vi "RTS Macro Filter Defrost Cycle.vi"(0 "Refrigeration Full Data":T1, 5 "Refrigeration Core Stats Input":T2 {"Average Compressor Cycle Time (Min)" format="%0.2f"; "Average Compressor Power (W)" format="%0.2f"; "Power Start Time (sec)" format="%<%H:%M:%S>t"; "Power End time (sec)" format="%<%H:%M:%S>t"; "Average Defrost Power (W)" format="%0.2f"}, 11 "Error In":errorcluster, 12 "Average Compressor Power (Lower)":dbl=10.0 format="%#_13g") -> (4 "Refrigeration Full Data Output":T1, 6 "Refrigeration Core Stats":T2 {"Average Compressor Cycle Time (Min)" format="%0.2f"; "Average Compressor Power (W)" format="%0.2f"; "Power Start Time (sec)" format="%<%H:%M:%S>t"; "Power End time (sec)" format="%<%H:%M:%S>t"; "Average Defrost Power (W)" format="%0.2f"}, 15 "Error Out":errorcluster)   [LabVIEW 2016]
uses:
  Type Definitions/RTS Macro Refrigeration Core Stats.ctl
  Type Definitions/RTS Macro Full Data.ctl
panel:
  out "Power Compressor Run 2":cluster{dbl[], dbl[]}(graph)
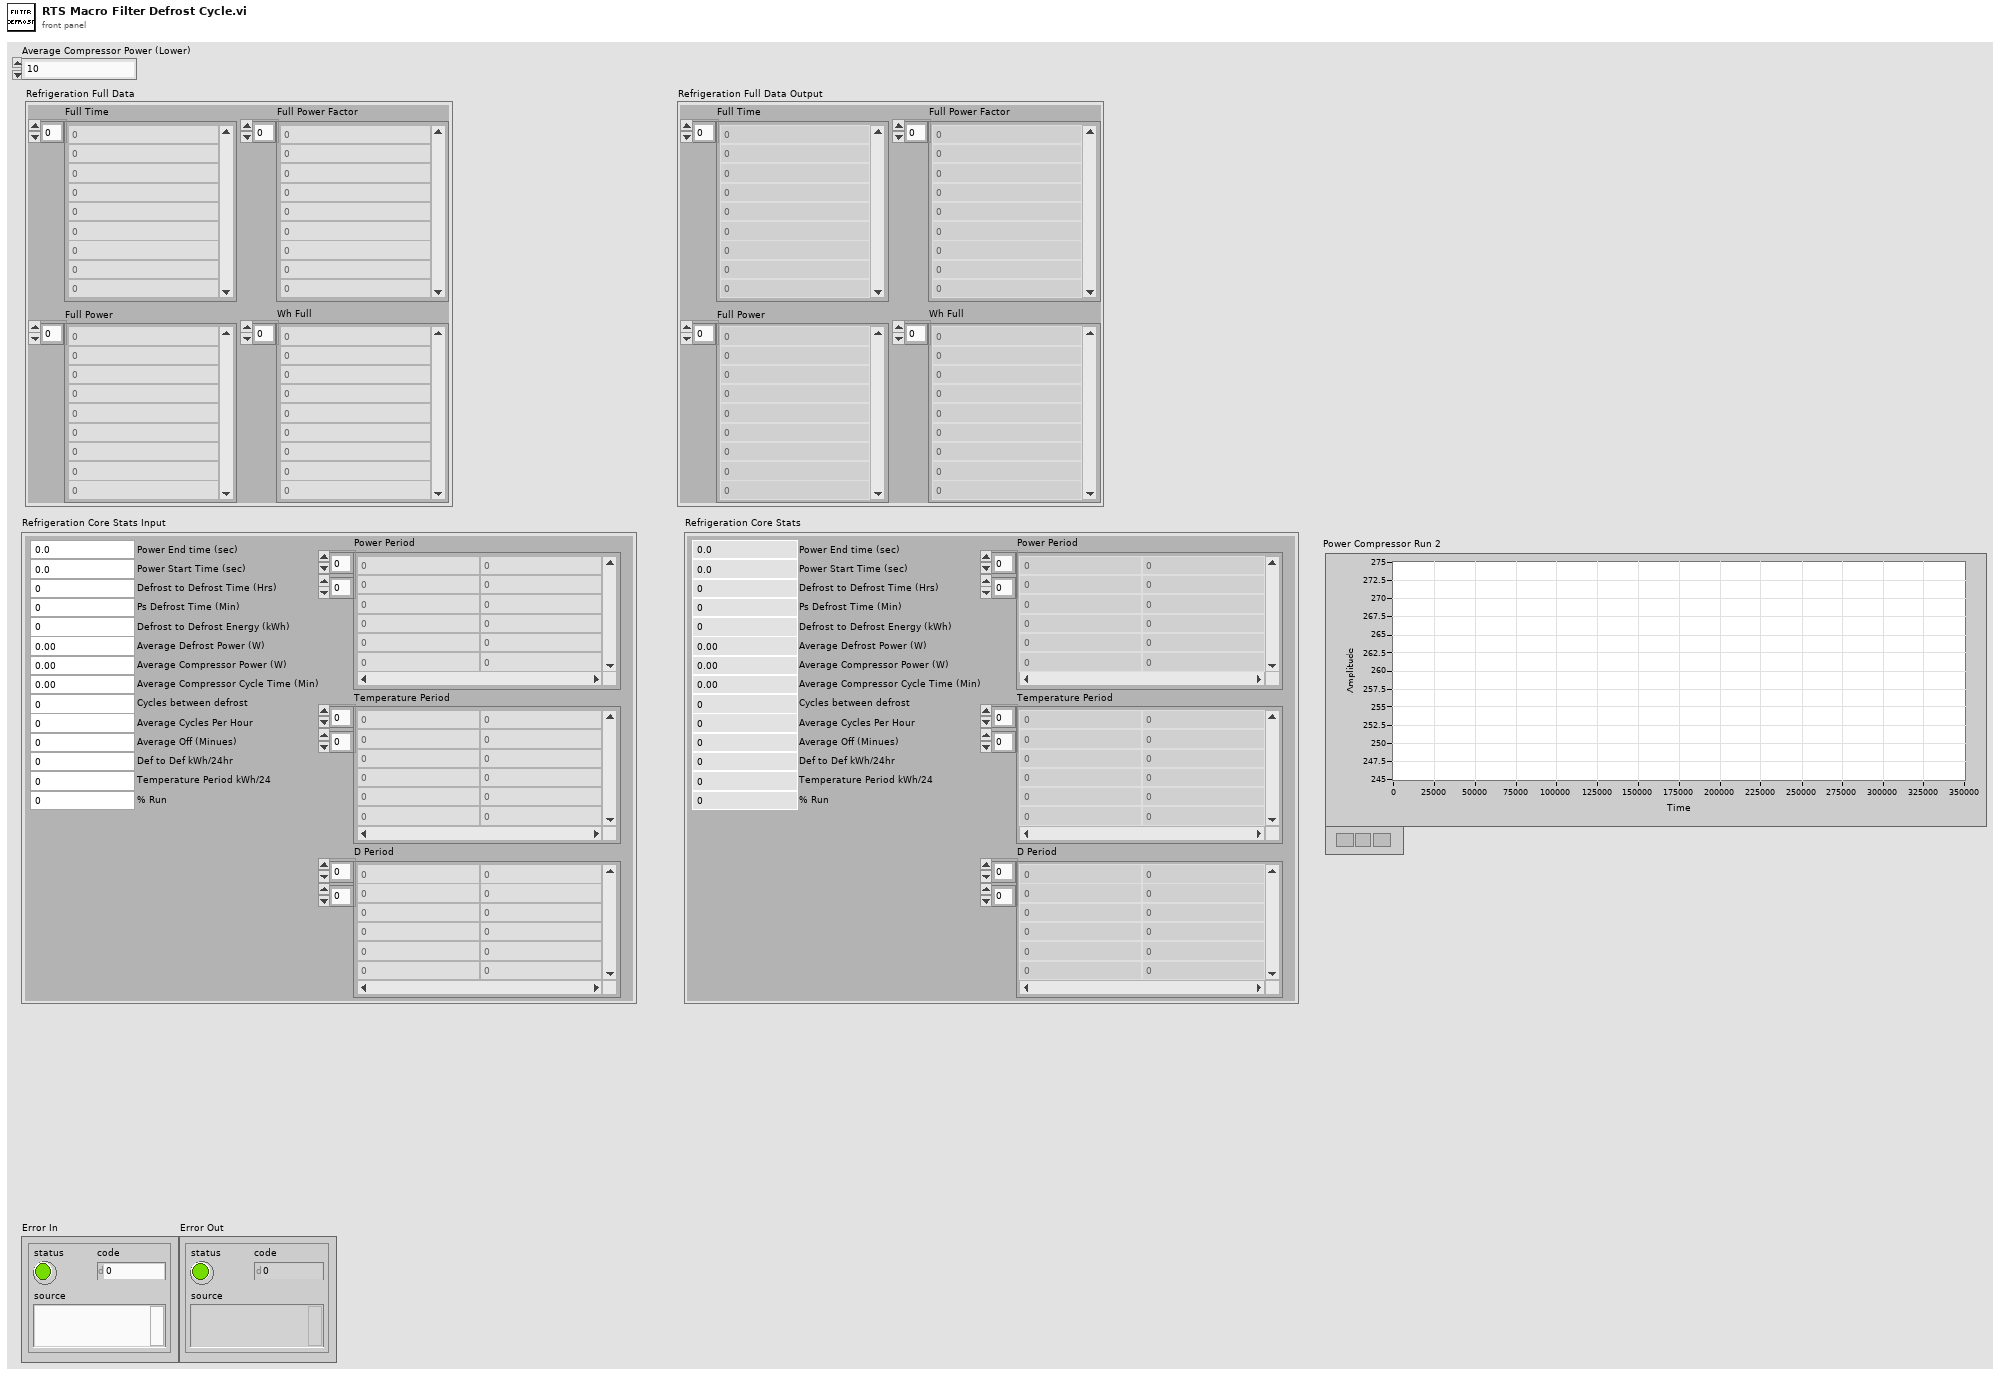
[diagram p1: front panel]
types:
  T1 = typedef "RTS Macro Full Data.ctl" = cluster{"Full Time":dbl[], "Full Power Factor":dbl[], "Full Power":dbl[], "Wh Full":dbl[]}
  T2 = typedef "RTS Macro Refrigeration Core Stats.ctl" = cluster{"Average Defrost Power (W)":dbl, "Power End time (sec)":dbl, "Power Start Time (sec)":dbl, "Defrost to Defrost Time (Hrs)":dbl, "Ps Defrost Time (Min)":dbl, "Defrost to Defrost Energy (kWh)":dbl, "Average Compressor Power (W)":dbl, "Average Compressor Cycle Time (Min)":dbl, "Power Period":dbl[][], "Cycles between defrost":i32, "Average Cycles Per Hour":dbl, "Average Off (Minues)":dbl, "Def to Def kWh/24hr":dbl, "Temperature Period kWh/24":dbl, "% Run":dbl, "Temperature Period":dbl[][], "D Period":dbl[][]}
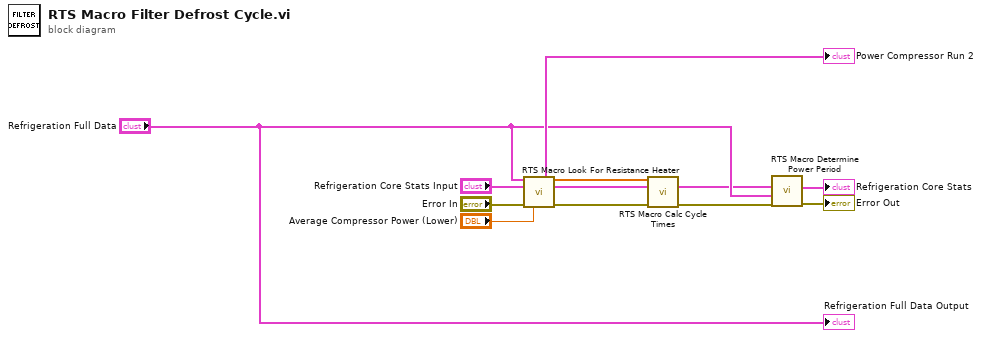
[diagram p0: block diagram]
diagram:
  n1 = call "RTS Macro Look For Resistance Heater.vi"("Refrigeration Full Data Output"="Refrigeration Full Data", "Refrigeration Core Stats Input"="Refrigeration Core Stats Input", "Error In"="Error In", "Average Compressor Power (Lower)"="Average Compressor Power (Lower)") -> ("Power Compressor Run 2"=→"Power Compressor Run 2":cluster{dbl[], dbl[]}, "Time Array"=w7:dbl[], "Refrigeration Core Stats Output"=w5:T2, "Error Out"=w9:errorcluster)  [unwired: 8 in]
  n2 = call "RTS Macro Calc Cycle Times.vi"("Time"=w7, "Refrigeration Core Stats Input"=w5, "Error In"=w9) -> ("Refrigeration Core Stats Output"=w2:T2, "Error Out"=w4:errorcluster)  [unwired: 8 in, 3 out]
  n3 = call "RTS Macro Determine Power Period.vi"("Refrigeration Core Stats Input"=w2, "Refrigeration Full Data"="Refrigeration Full Data", "Error In"=w4) -> ("Refrigeration Core Stats Output"=→"Refrigeration Core Stats":T2, "Error Out"=→"Error Out":errorcluster)  [unwired: 5 in, 1 out]
  "Refrigeration Full Data Output" <- "Refrigeration Full Data"
